vi "Merge.vi"(9 "new gesture in":refnum<class "Gesture.lvclass">, 11 "gesture in":refnum<class "Gesture.lvclass">) -> (0 "merged?":bool, 3 "gesture out":refnum<class "Gesture.lvclass">)   [LabVIEW 2023, in "Gesture.lvclass"]
doc: "Merge two gestures into a single gesture."
uses:
  Gesture.lvclass
  Gesture.lvclass/Gesture.ctl
  Gesture Enum.ctl
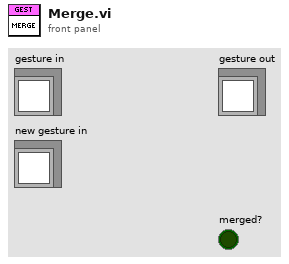
[diagram p1: front panel]
types:
  T1 = typedef "Gesture.lvclass/Gesture Enum.ctl" = enum16{"None", "Stop", "Tap", "Press", "Pan Start", "Pan Continue", "Pan End", "Pinch Open", "Pinch Close", "Double Tap"}
  T2 = typedef "LVPoint32TypeDef.ctl" = cluster{"Horizontal":i32, "Vertical":i32}
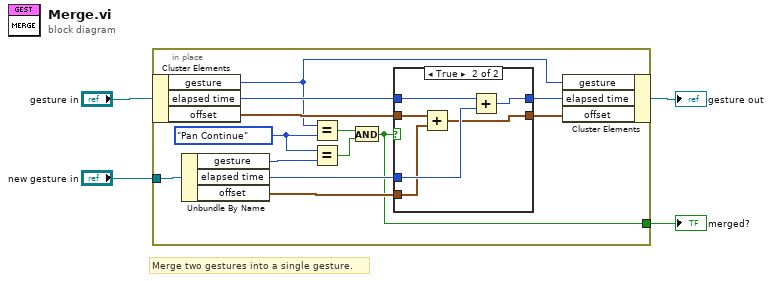
[diagram p0: block diagram]
diagram:
  # "Merge two gestures into a single gesture."
  n1 = in-place {
    in-place-border: "new gesture in" -> [w17]
    in-place-border: [w10] -> w2
    w6 = Gesture_Enum."Pan Continue" ("x")
    n2 = in-place-cluster #1("gesture in") -> ("gesture"=w5:T1, "elapsed time"=w16:u32, "offset"=w13:T2)
    n3 = Unbundle By Name(w17) -> ("gesture"=w9:T1, "elapsed time"=w14:u32, "offset"=w12:T2)
    n4 = Equal?(x=w5, y=w6) -> (x = y?=w7:bool)
    n5 = Equal?(x=w6, y=w9) -> (x = y?=w8:bool)
    n6 = And(x=w7, y=w8) -> (x .and. y?=w10:bool)
    n7 = case shown="True" w10 {
      tunnel: w16 -> [w19 w25]
      tunnel: [w19 w24] -> w15
      tunnel: w14 -> [_ w23]
      tunnel: w13 -> [w18 w22]
      tunnel: w12 -> [_ w21]
      tunnel: [w18 w20] -> w11
      frame False {
      }
      frame True {
        n8 = Add(x=w22, y=w21) -> (x+y=w20:T2)
        n9 = Add(x=w25, y=w23) -> (x+y=w24:u32)
      }
    }
    n10 = in-place-cluster #1("gesture"=w5, "elapsed time"=w15, "offset"=w11) -> (→"gesture out":refnum<class "Gesture.lvclass">)
  }
  "merged?" <- w2
